vi "Set Width.vi"(8 "error in (no error)":errorcluster caption="错误输入（无错误）", 10 "Width":i32, 11 "ToolStripLabel 输入":refnum<class "ToolStripLabel.lvclass"> caption="DNL_LabVIEW Object in") -> (0 "error out":errorcluster caption="错误输出", 3 "ToolStripLabel 输出":refnum<class "ToolStripLabel.lvclass"> caption="DNL_LabVIEW Object out")   [LabVIEW 2013, in "ToolStripLabel.lvclass"]
uses:
  ToolStripLabel.lvclass
  ToolStripLabel.lvclass/ToolStripLabel.ctl
  System.Windows.Forms
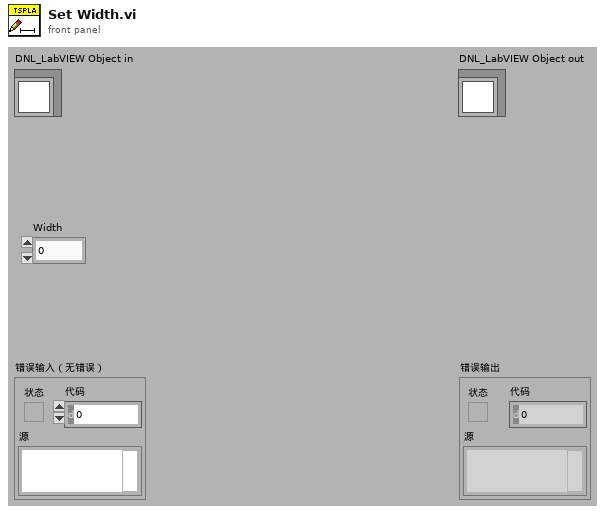
[diagram p1: front panel]
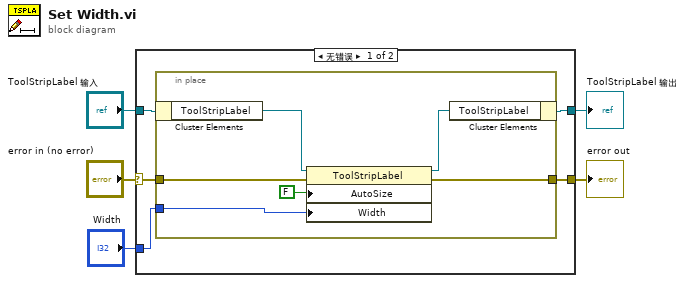
[diagram p0: block diagram]
diagram:
  n1 = case shown="无错误" "error in (no error)" {
    selector: "error in (no error)" -> [w7 w18]
    tunnel: [w6 w18] -> w4
    tunnel: [w8 w17] -> w2
    tunnel: "ToolStripLabel 输入" -> [w10 w17]
    tunnel: "Width" -> [w9 _]
    frame No Error {
      n2 = in-place {
        in-place-border: w9 -> [w15]
        in-place-border: w7 -> [w12]
        in-place-border: [w11] -> w6
        n3 = in-place-cluster #1(w10) -> ("ToolStripLabel"=w14:refnum<k24>)
        n4 = property class="ToolStripLabel"(reference=w14, error in=w12, "AutoSize"=FALSE, "Width"=w15) -> (reference out=w13:refnum<k24>, error out=w11:errorcluster)
        n5 = in-place-cluster #1("ToolStripLabel"=w13) -> (w8:refnum<class "ToolStripLabel.lvclass">)
      }
    }
    frame Error {
    }
  }
  "error out" <- w4
  "ToolStripLabel 输出" <- w2
